vi "E2 Data Logger.vi"(7 "refnum in":refnum<file>) -> (3 "refnum out":refnum<file>)   [LabVIEW 2015]
uses:
  <vilib>/Rock Robotics/WPI/DriverStation/WPI_DriverStationRobotMode2.ctl
  Robot Global Data.vi
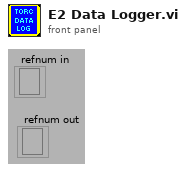
[diagram p1: front panel]
types:
  T1 = typedef "WPI_DriverStationRobotMode2.ctl" = enum16{"Autonomous Disabled", "Autonomous Enabled", "Teleop Disabled", "Teleop Enabled", "Disconnected", "Finish", "Test Disabled", "Test Enabled", "Emergency Stopped"}
  T2 = enum16{"CW_Fast", "CW_Slow", "CCW_Fast", "CCW_Slow", "Straight", "WaitingForStraight", "Rotate_Move"}
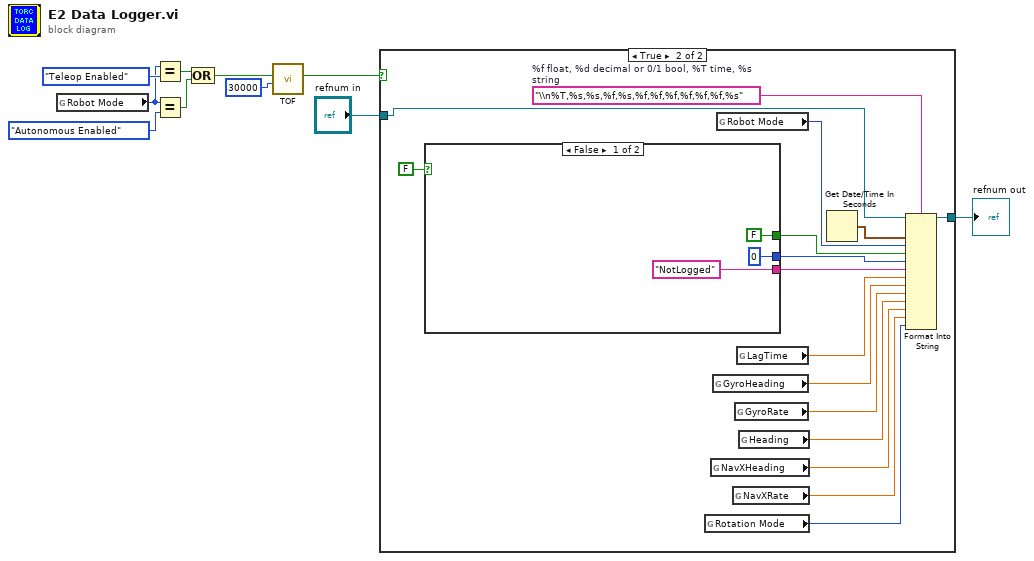
[diagram p0: block diagram]
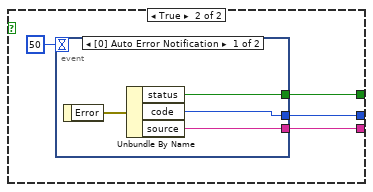
[diagram p3: hidden frame]
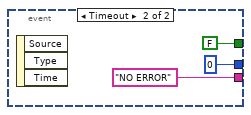
[diagram p4: hidden frame]
diagram:
  n1 = global read "Robot Global Data.vi" "Robot Mode"() -> (w4:T1)
  n2 = Equal?(x=w4, y=WPI_DriverStationRobotMode2."Teleop Enabled") -> (x = y?=w6:bool)
  n3 = Equal?(x=w4, y=WPI_DriverStationRobotMode2."Autonomous Enabled") -> (x = y?=w5:bool)
  n4 = Compound Arithmetic op=OR(w6, w5) -> (w3:bool)
  n5 = call "TOF.vi"("Delay (ms)"=u32 30000, "Input"=w3) -> ("Output"=w2:bool)  [unwired: 9 in]
  n6 = case shown="True" w2 {
    tunnel: [w11 w27] -> w10
    tunnel: "refnum in" -> [w11 w23]
    frame False {
    }
    frame True {
      w24 = "\\n%T,%s,%s,%f,%s,%f,%f,%f,%f,%f,%f,%s"  # %f float, %d decimal or 0/1 bool, %T time, %s string
      n7 = case shown="False" FALSE {
        tunnel: [FALSE ("status") w33] -> w15
        tunnel: [0 ("code") w32] -> w14
        tunnel: ["NotLogged" ("source") w31] -> w13
        frame False {
        }
        frame True {
          n8 = event shown="[0] Auto Error Notification" {
            selector: _ -> [_ _]
            dyn-events: _ -> [_ _]
            timeout: 50 -> [_ _]
            tunnel: [w37 "NO ERROR" ("source")] -> w31
            tunnel: [w36 0 ("code")] -> w32
            tunnel: [w35 FALSE ("status")] -> w33
            event Auto Error Notification {
              n9 = event-data() -> ("Error"=w38:errorcluster)  [unwired: 1 in]
              n10 = Unbundle By Name(w38) -> ("status"=w35:bool, "code"=w36:i32, "source"=w37:string)
            }
            event Timeout {
              n11 = event-data() -> ()  [unwired: 1 in, 3 out]
            }
          }
        }
      }
      n12 = global read "Robot Global Data.vi" "Rotation Mode"() -> (w16:T2)
      n13 = global read "Robot Global Data.vi" "NavXHeading"() -> (w18:dbl)
      n14 = global read "Robot Global Data.vi" "GyroHeading"() -> (w21:dbl)
      n15 = global read "Robot Global Data.vi" "Robot Mode"() -> (w25:T1)
      n16 = global read "Robot Global Data.vi" "NavXRate"() -> (w17:dbl)
      n17 = global read "Robot Global Data.vi" "GyroRate"() -> (w20:dbl)
      n18 = global read "Robot Global Data.vi" "LagTime"() -> (w22:dbl)
      n19 = global read "Robot Global Data.vi" "Heading"() -> (w19:dbl)
      n20 = Get Date/Time In Seconds() -> (seconds since 1Jan1904=w26:timestamp)
      n21 = Format Into String(format string=w24, initial string=w23, w26, w25, w15, w14, w13, w22, w21, w20, w19, w18, w17, w16) -> (resulting string=w27:refnum<file>)  [unwired: 1 in, 1 out]
    }
  }
  "refnum out" <- w10
